vi "AD5781StayInState.vi"(2 "lastDacState":T1) -> (16 "newDacState":T1)   [LabVIEW 2014]
uses:
  Controls/DacState.ctl
  <vilib>/rvi/Emulation/niFpgaGetClockAttributes.vi
  <vilib>/rvi/Emulation/niFpgaSctlEmulationGetInTimedLoop.vi
  <vilib>/rvi/Emulation/niFpgaEmulationReportErrorSimple.vi
  Code/FPGA SPI_Globals.vi
  <vilib>/rvi/Emulation/niFpgaCriticalErrorInLSC.vi
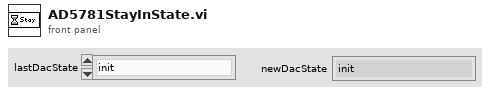
[diagram p1: front panel]
types:
  T1 = typedef "DacState.ctl" = enum16{"init", "idle", "setVolt", "error"}
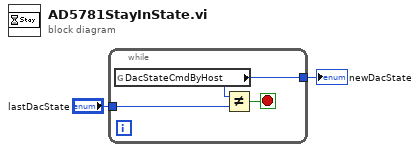
[diagram p0: block diagram]
diagram:
  n1 = while {
    tunnel: "lastDacState" -> [w5]
    tunnel: [w3] -> w1
    stop <- w4 stop-if-true
    n2 = global read "FPGA SPI_Globals.vi" "DacStateCmdByHost"() -> (w3:T1)
    n3 = Not Equal?(x=w3, y=w5) -> (x != y?=w4:bool)
  }
  "newDacState" <- w1
